vi "ReadFile.vi"() -> ()   [LabVIEW 2014]
panel:
  in  "name or relative path":string="FileIO.txt"
  in  "base path":path
  out "text from file":string
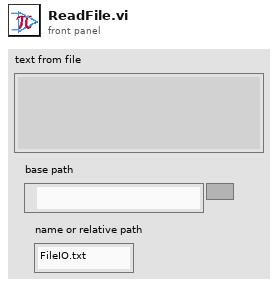
[diagram p1: front panel]
types:
  T1 = enum16{"open", "replace", "create", "open or create", "replace or create", "replace or create with confirmation"}
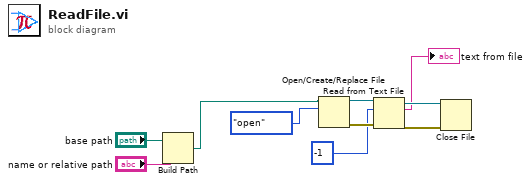
[diagram p0: block diagram]
diagram:
  n1 = Build Path(base path="base path", name or relative path="name or relative path") -> (appended path=w6:path)
  n2 = Open/Create/Replace File(file path (use dialog)=w6, operation (0:open)=T1."open") -> (refnum out=w4:refnum<file>, error out=w8:errorcluster)  [unwired: 4 in, 1 out]
  n3 = Read from Text File(file (use dialog)=w4, count=-1, error in=w8) -> (refnum out=w3:refnum<file>, text=→"text from file":string, error out=w7:errorcluster)  [unwired: 1 in, 1 out]
  n4 = Close File(refnum=w3, error in=w7) -> ()  [unwired: 2 out]
